vi "DAQ setup.vi"(0 "Vx_min":dbl, 1 "Vx_max":dbl, 2 "数组":waveform(dbl)[](array[waveform]), 5 "rate":dbl, 7 "physical channels write":tag, 9 "Timing source":tag, 12 "sample mode":i32, 13 "physical channels read":tag, 14 "Number of samples per channel":i32) -> (4 "Writing task out":refnum<k21>, 6 "Reading task out":refnum<k21>, 15 "错误输出":errorcluster)   [LabVIEW 2013]
uses:
  <vilib>/DAQmx/write.llb/DAQmx Write (Analog 1D Wfm NChan NSamp).vi
  <vilib>/DAQmx/create/channels.llb/DAQmx Create Channel (AI-Voltage-Basic).vi
  <vilib>/DAQmx/configure/timing.llb/DAQmx Timing (Sample Clock).vi
  <vilib>/DAQmx/configure/trigger.llb/DAQmx Start Trigger (Analog Edge).vi
  <vilib>/DAQmx/create/channels.llb/DAQmx Create Channel (AO-Voltage-Basic).vi
  <vilib>/DAQmx/miscellaneous.llb/DAQmx Fill In Error Info.vi
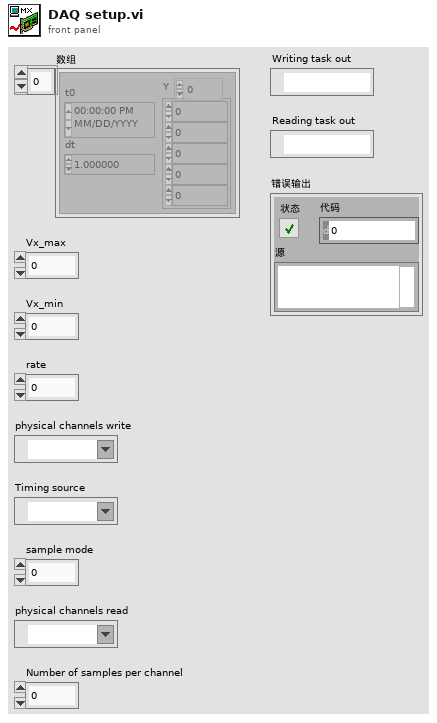
[diagram p1: front panel]
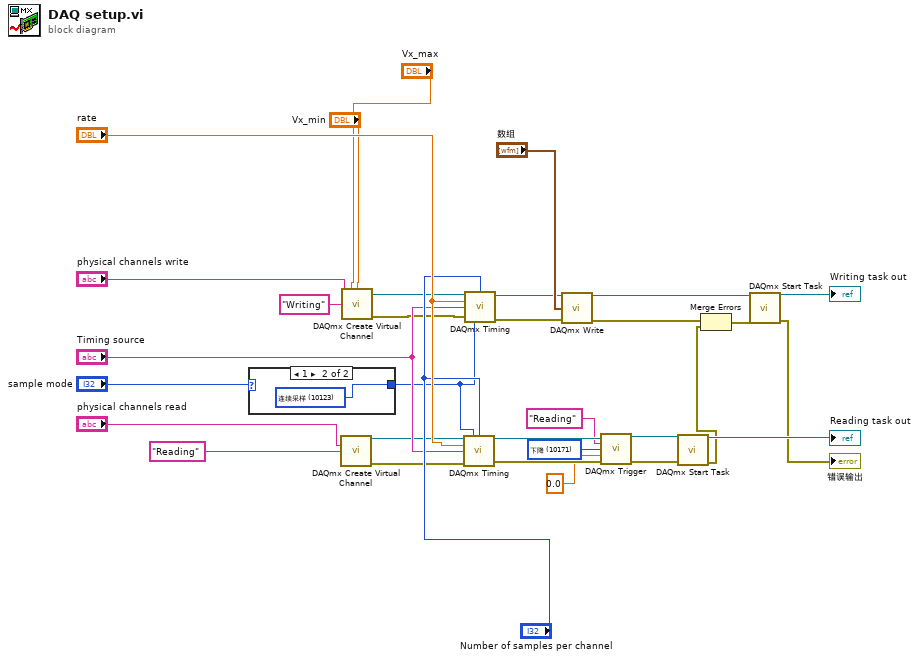
[diagram p0: block diagram]
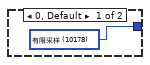
[diagram p2: hidden frame]
diagram:
  w28 = 10171 items=["上升"=10280, "下降"=10171] ("slope")
  n1 = case shown="1" "sample mode" {
    tunnel: [w33 w34] -> w7
    frame 0, Default {
      w33 = 10178 items=["有限采样"=10178, "连续采样"=10123, "硬件定时单点"=12522] ("sample mode")
    }
    frame 1 {
      w34 = 10123 items=["有限采样"=10178, "连续采样"=10123, "硬件定时单点"=12522] ("sample mode")
    }
  }
  n2 = call-poly <vilib>:"DAQmx Create Virtual Channel.vi"("physical channels"="physical channels read", "name to assign"="Reading") -> ("task out"=w9:refnum<k21>, "error out"=w10:errorcluster)  [unwired: 12 in]
  n3 = call-poly <vilib>:"DAQmx Create Virtual Channel.vi"("maximum value"="Vx_max", "minimum value"="Vx_min", "physical channels"="physical channels write", "name to assign"="Writing") -> ("task out"=w15:refnum<k21>, "error out"=w16:errorcluster)  [unwired: 10 in]
  n4 = call-poly <vilib>:"DAQmx Timing.vi"("task/channels in"=w9, "sample mode"=w7, "samples per channel"="Number of samples per channel", "rate"="rate", "source"="Timing source", "error in"=w10) -> ("task out"=w30:refnum<k21>, "error out"=w31:errorcluster)  [unwired: 8 in]
  n5 = call-poly <vilib>:"DAQmx Timing.vi"("task/channels in"=w15, "sample mode"=w7, "samples per channel"="Number of samples per channel", "rate"="rate", "source"="Timing source", "error in"=w16) -> ("task out"=w11:refnum<k21>, "error out"=w12:errorcluster)  [unwired: 8 in]
  n6 = call-poly <vilib>:"DAQmx Write.vi"("task/channels in"=w11, "data"="数组", "error in"=w12) -> ("task out"=w23:refnum<k21>, "error out"=w4:errorcluster)  [unwired: 10 in, 1 out]
  n7 = call-poly <vilib>:"DAQmx Trigger.vi"("task/channels in"=w30, "source"="Reading", "slope"=w28, "level"=0.0, "error in"=w31) -> ("task out"=w32:refnum<k21>, "error out"=w5:errorcluster)  [unwired: 9 in]
  n8 = call <vilib>:"DAQmx Start Task.vi"("task/channels in"=w32, "error in"=w5) -> ("task out"=→"Reading task out":refnum<k21>, "error out"=w2:errorcluster)  [unwired: 12 in]
  n9 = Merge Errors(w4, w2) -> (w3:errorcluster)
  n10 = call <vilib>:"DAQmx Start Task.vi"("task/channels in"=w23, "error in"=w3) -> ("task out"=→"Writing task out":refnum<k21>, "error out"=→"错误输出":errorcluster)  [unwired: 12 in]
